vi "OE2052_Configure Auto_Setting.vi"(7 "OE2052_Auto Setting":T1={"Auto Range"=FALSE, "Auto Offest"=FALSE, "Auto Phase"=FALSE, "channel"=1} {"channel" items=["A"=1, "B"=2]}, 8 "Error in (no error)":errorcluster caption="error out（no error）", 9 "Remote Mode":u16(ring) items=["USB"=0, "RS232"=1, "Ethernet"=3], 10 "Connection ID in":refnum<k5>, 11 "VISA resource name":refnum<visa-resource-name>) -> (0 "Error out":errorcluster caption="error out", 1 "Output String":string, 2 "Connection ID out":refnum<k5>, 3 "VISA resource  out":refnum<visa-resource-name>)   [LabVIEW 2011]
panel:
  out "channel":u16
  out "字符串":string
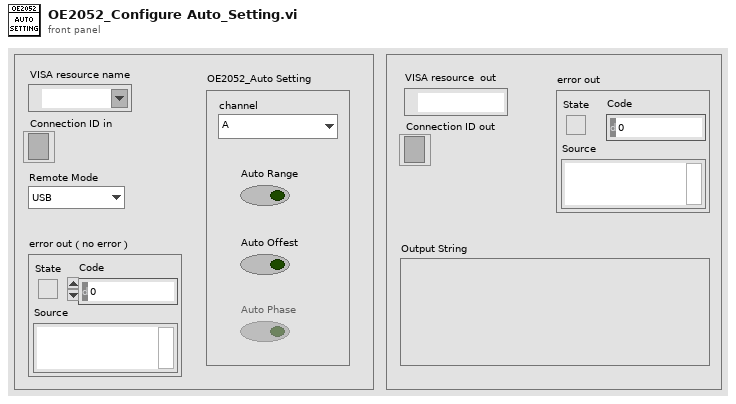
[diagram p1: front panel]
types:
  T1 = cluster{"Auto Range":bool, "Auto Offest":bool, "Auto Phase":bool, "channel":u16}
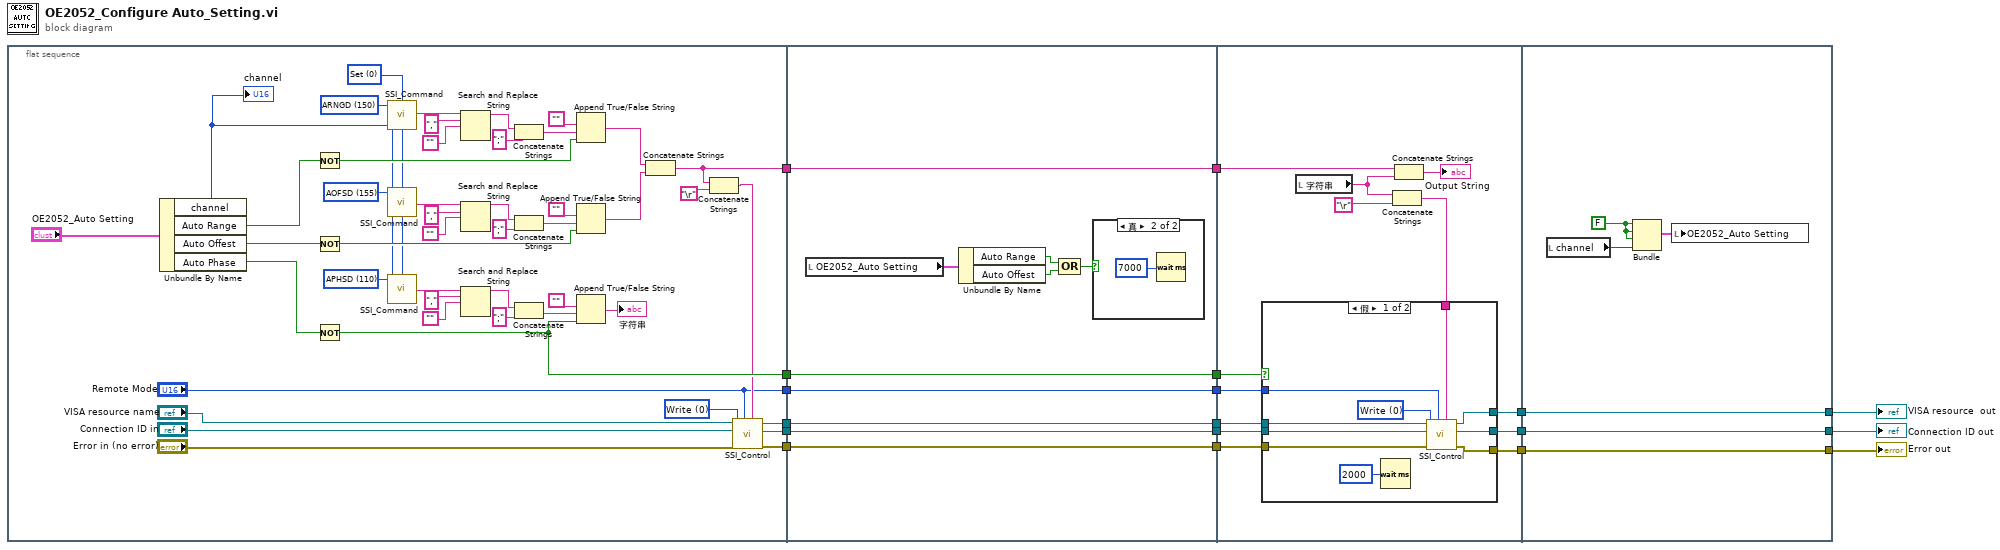
[diagram p0: block diagram]
diagram:
  n1 = flat-sequence {
    tunnel: [w61] -> w18
    tunnel: [w60] -> w17
    tunnel: [w59] -> w16
    tunnel: [w30] -> w11
    tunnel: [w25] -> w7
    tunnel: ["Remote Mode"] -> w5
    tunnel: w18 -> [w75]
    tunnel: w17 -> [w74]
    tunnel: w16 -> [w73]
    tunnel: [w75] -> w15
    tunnel: [w74] -> w14
    tunnel: [w73] -> w13
    tunnel: [w68] -> w12
    tunnel: w11 -> [w68]
    tunnel: w7 -> [w67]
    tunnel: [w67] -> w6
    tunnel: w5 -> [w66]
    tunnel: [w66] -> w4
    tunnel: w15 -> [w87]
    tunnel: w14 -> [w88]
    tunnel: w13 -> [w86]
    tunnel: w12 -> [w89]
    tunnel: w6 -> [w81]
    tunnel: w4 -> [w80]
    tunnel: [w85] -> w3
    tunnel: [w84] -> w2
    tunnel: [w83] -> w1
    tunnel: [w106] -> w8
    tunnel: [w107] -> w9
    tunnel: [w108] -> w10
    tunnel: w3 -> [w108]
    tunnel: w2 -> [w107]
    tunnel: w1 -> [w106]
    frame #0 {
      w20 = u16 110 items=["ISRC", "IGND", "ICPL", "ILIN", "PHAS", "FMOD", "RSLP", "FREQ", "SWPT", "SLLM", "SULM", "SSLL", "SSLG", "STLM", "SWRM", "IRNG", "SENS", "RMOD", "OFLT", "OFSL", "SYNC", "DMOD", "HARM", "DARB", "SWVT", "SLVL", "SVLL", "SVUL", "SVSL", "SVSG", "SVTM", "SVRM", "RALL", "SNAP", "OUTP", "OAUX", "COUT", "CAUX", "COFP", "CEXP", "FPOP", "OEXP", "*IDN", "*RST", "OVLD", "INOV", "GNOV", "*PLL", "SSET", "RSET", "AGAN", "APHS", "ARSV", "ASCL", "EQCD", "EQCS", "SPED", "SRAT", "SLEN", "SSLE", "STRG", "SPRM", "STRD", "PAUS", "REST", "SPTS", "TRCA", "TEMP", "RSTU", "INHZ", "DEQU", "SADD", "ARNG", "CSPE", "ISRCD", "IGNDD", "ICPLD", "ILIND", "PHASD", "FMODD", "RSLPD", "FREQD", "SWPTD", "SLLMD", "SULMD", "SSLLD", "SSLGD", "STLMD", "SWRMD", "SENSD", "RMODD", "OFLTD", "OFSLD", "SYNCD", "HARMD", "EQCDD", "EQCSD", "SNAPD", "OUTPD", "SWVTD", "SLVLD", "SVLLD", "SVULD", "SVSLD", "SVSGD", "SVTMD", "SVRMD", "SVDCD", "ARSVD", "AGAND", "APHSD", "ASCLD", "FPOPD", "CAUXD", "OEXPD", "SPEDD", "SRATD", "SLEND", "SSLED", "STRGD", "SPRMD", "STRDD", "PAUSD", "RESTD", "SPTSD", "TRCAD", "*IDND", "*RSTD", "INOVD", "GNOVD", "*PLLD", "SSETD", "RSETD", "RALLD", "NIPA", "NSMA", "NGWA", "NMAC", "NMOD", "TRIG", "TRCB", "INHZD", "ISAMD", "IRAGD", "RRAGD", "SOFFD", "DMODD", "COUTD", "COFPD", "CEXPD", "ARNGD", "OAUXD", "TRIM", "SUITD", "SNHZD", "AOFSD"] ("Command Type")
      w21 = u16 155 items=["ISRC", "IGND", "ICPL", "ILIN", "PHAS", "FMOD", "RSLP", "FREQ", "SWPT", "SLLM", "SULM", "SSLL", "SSLG", "STLM", "SWRM", "IRNG", "SENS", "RMOD", "OFLT", "OFSL", "SYNC", "DMOD", "HARM", "DARB", "SWVT", "SLVL", "SVLL", "SVUL", "SVSL", "SVSG", "SVTM", "SVRM", "RALL", "SNAP", "OUTP", "OAUX", "COUT", "CAUX", "COFP", "CEXP", "FPOP", "OEXP", "*IDN", "*RST", "OVLD", "INOV", "GNOV", "*PLL", "SSET", "RSET", "AGAN", "APHS", "ARSV", "ASCL", "EQCD", "EQCS", "SPED", "SRAT", "SLEN", "SSLE", "STRG", "SPRM", "STRD", "PAUS", "REST", "SPTS", "TRCA", "TEMP", "RSTU", "INHZ", "DEQU", "SADD", "ARNG", "CSPE", "ISRCD", "IGNDD", "ICPLD", "ILIND", "PHASD", "FMODD", "RSLPD", "FREQD", "SWPTD", "SLLMD", "SULMD", "SSLLD", "SSLGD", "STLMD", "SWRMD", "SENSD", "RMODD", "OFLTD", "OFSLD", "SYNCD", "HARMD", "EQCDD", "EQCSD", "SNAPD", "OUTPD", "SWVTD", "SLVLD", "SVLLD", "SVULD", "SVSLD", "SVSGD", "SVTMD", "SVRMD", "SVDCD", "ARSVD", "AGAND", "APHSD", "ASCLD", "FPOPD", "CAUXD", "OEXPD", "SPEDD", "SRATD", "SLEND", "SSLED", "STRGD", "SPRMD", "STRDD", "PAUSD", "RESTD", "SPTSD", "TRCAD", "*IDND", "*RSTD", "INOVD", "GNOVD", "*PLLD", "SSETD", "RSETD", "RALLD", "NIPA", "NSMA", "NGWA", "NMAC", "NMOD", "TRIG", "TRCB", "INHZD", "ISAMD", "IRAGD", "RRAGD", "SOFFD", "DMODD", "COUTD", "COFPD", "CEXPD", "ARNGD", "OAUXD", "TRIM", "SUITD", "SNHZD", "AOFSD"] ("Command Type")
      w23 = u16 150 items=["ISRC", "IGND", "ICPL", "ILIN", "PHAS", "FMOD", "RSLP", "FREQ", "SWPT", "SLLM", "SULM", "SSLL", "SSLG", "STLM", "SWRM", "IRNG", "SENS", "RMOD", "OFLT", "OFSL", "SYNC", "DMOD", "HARM", "DARB", "SWVT", "SLVL", "SVLL", "SVUL", "SVSL", "SVSG", "SVTM", "SVRM", "RALL", "SNAP", "OUTP", "OAUX", "COUT", "CAUX", "COFP", "CEXP", "FPOP", "OEXP", "*IDN", "*RST", "OVLD", "INOV", "GNOV", "*PLL", "SSET", "RSET", "AGAN", "APHS", "ARSV", "ASCL", "EQCD", "EQCS", "SPED", "SRAT", "SLEN", "SSLE", "STRG", "SPRM", "STRD", "PAUS", "REST", "SPTS", "TRCA", "TEMP", "RSTU", "INHZ", "DEQU", "SADD", "ARNG", "CSPE", "ISRCD", "IGNDD", "ICPLD", "ILIND", "PHASD", "FMODD", "RSLPD", "FREQD", "SWPTD", "SLLMD", "SULMD", "SSLLD", "SSLGD", "STLMD", "SWRMD", "SENSD", "RMODD", "OFLTD", "OFSLD", "SYNCD", "HARMD", "EQCDD", "EQCSD", "SNAPD", "OUTPD", "SWVTD", "SLVLD", "SVLLD", "SVULD", "SVSLD", "SVSGD", "SVTMD", "SVRMD", "SVDCD", "ARSVD", "AGAND", "APHSD", "ASCLD", "FPOPD", "CAUXD", "OEXPD", "SPEDD", "SRATD", "SLEND", "SSLED", "STRGD", "SPRMD", "STRDD", "PAUSD", "RESTD", "SPTSD", "TRCAD", "*IDND", "*RSTD", "INOVD", "GNOVD", "*PLLD", "SSETD", "RSETD", "RALLD", "NIPA", "NSMA", "NGWA", "NMAC", "NMOD", "TRIG", "TRCB", "INHZD", "ISAMD", "IRAGD", "RRAGD", "SOFFD", "DMODD", "COUTD", "COFPD", "CEXPD", "ARNGD", "OAUXD", "TRIM", "SUITD", "SNHZD", "AOFSD"] ("Command Type")
      w22 = u16 0 items=["Set", "Query"] ("Opera")
      w62 = u16 0 items=["Write", "Read"] ("Control")
      n2 = Unbundle By Name("OE2052_Auto Setting") -> ("channel"=w19:u16, "Auto Range"=w31:bool, "Auto Offest"=w34:bool, "Auto Phase"=w35:bool)
      "channel" <- w19
      n3 = Not(x=w31) -> (.not. x?=w32:bool)
      n4 = Not(x=w34) -> (.not. x?=w33:bool)
      n5 = Not(x=w35) -> (.not. x?=w30:bool)
      n6 = call "SSI_Command.vi"("Opera"=w22, "channel"=w19, "Command Type"=w23) -> ("Output string"=w38:string)  [unwired: 1 in]
      n7 = call "SSI_Command.vi"("Opera"=w22, "channel"=w19, "Command Type"=w21) -> ("Output string"=w40:string)  [unwired: 1 in]
      n8 = call "SSI_Command.vi"("Opera"=w22, "channel"=w19, "Command Type"=w20) -> ("Output string"=w39:string)  [unwired: 1 in]
      n9 = Search and Replace String(input string=w38, search string="," ("搜索字符串"), replace string="") -> (result string=w50:string)  [unwired: 5 in, 3 out]
      n10 = Search and Replace String(input string=w40, search string="," ("搜索字符串"), replace string="") -> (result string=w47:string)  [unwired: 5 in, 3 out]
      n11 = Search and Replace String(input string=w39, search string="," ("搜索字符串"), replace string="") -> (result string=w44:string)  [unwired: 5 in, 3 out]
      n12 = Concatenate Strings(w50, ";") -> (w43:string)
      n13 = Concatenate Strings(w47, ";") -> (w42:string)
      n14 = Concatenate Strings(w44, ";") -> (w41:string)
      n15 = Append True/False String(1:w32, 2:w43, 3:"") -> (0:w29:string)  [unwired: 1 in]
      n16 = Append True/False String(1:w33, 2:w42, 3:"") -> (0:w28:string)  [unwired: 1 in]
      n17 = Append True/False String(1:w30, 2:w41, 3:"") -> (0:→"字符串":string)  [unwired: 1 in]
      n18 = Concatenate Strings(w29, w28) -> (w25:string)
      n19 = Concatenate Strings(w25, "\r") -> (w26:string)
      n20 = call "SSI_Control.vi"("Write Buffer"=w26, "Remote Mode"="Remote Mode", "Error in (no error)"="Error in (no error)", "Control"=w62, "Connection ID in"="Connection ID in", "VISA resource name"="VISA resource name") -> ("Error out"=w59:errorcluster, "Connection ID out"=w61:refnum<k5>, "VISA resource  out"=w60:refnum<visa-resource-name>)  [unwired: 2 in, 1 out]
    }
    frame #1 {
      n21 = local read "OE2052_Auto Setting"() -> (w69:T1)
      n22 = Unbundle By Name(w69) -> ("Auto Range"=w71:bool, "Auto Offest"=w70:bool)
      n23 = Compound Arithmetic op=OR(w71, w70) -> (w72:bool)
      n24 = case shown="真" w72 {
        frame False {
        }
        frame True {
          n25 = Wait (ms)(milliseconds to wait=u32 7000 ("等待时间（毫秒）")) -> ()  [unwired: 1 out]
        }
      }
    }
    frame #2 {
      n26 = local read "字符串"() -> (w79:string)
      n27 = Concatenate Strings(w79, "\r") -> (w77:string)
      n28 = case shown="假" w89 {
        tunnel: w88 -> [w98 w102]
        tunnel: w87 -> [w97 w101]
        tunnel: w86 -> [w96 w100]
        tunnel: [w95 w100] -> w85
        tunnel: [w94 w101] -> w84
        tunnel: [w93 w102] -> w83
        tunnel: w77 -> [w91 _]
        tunnel: w80 -> [w90 _]
        frame False {
          w99 = u16 0 items=["Write", "Read"] ("Control")
          n29 = Wait (ms)(milliseconds to wait=u32 2000 ("等待时间（毫秒）")) -> ()  [unwired: 1 out]
          n30 = call "SSI_Control.vi"("Write Buffer"=w91, "Remote Mode"=w90, "Error in (no error)"=w96, "Control"=w99, "Connection ID in"=w97, "VISA resource name"=w98) -> ("Error out"=w95:errorcluster, "Connection ID out"=w94:refnum<k5>, "VISA resource  out"=w93:refnum<visa-resource-name>)  [unwired: 2 in, 1 out]
        }
        frame True {
        }
      }
      n31 = Concatenate Strings(w81, w79) -> (→"Output String":string)
    }
    frame #3 {
      w103 = FALSE
      n32 = local read "channel"() -> (w104:u16)
      n33 = Bundle(w103, w103, w103, "channel"=w104) -> (w105:cluster{bool, bool, bool, "channel":u16})  [unwired: 1 in]
      n34 = local write "OE2052_Auto Setting"(w105) -> ()
    }
  }
  "Error out" <- w10
  "Connection ID out" <- w9
  "VISA resource  out" <- w8
